vi "Get Tag.vi"(8 "error in (no error)":errorcluster, 11 "Item Configuration in":refnum<class "Item Configuration.lvclass">) -> (0 "error out":errorcluster, 2 "Project Info Tag":string, 3 "Item Configuration out":refnum<class "Item Configuration.lvclass">)   [LabVIEW 2013, in "Item Configuration.lvlib" / "Item Configuration.lvclass"]
uses:
  Item Configuration.lvclass
  Item Configuration.lvclass/Item Configuration.ctl
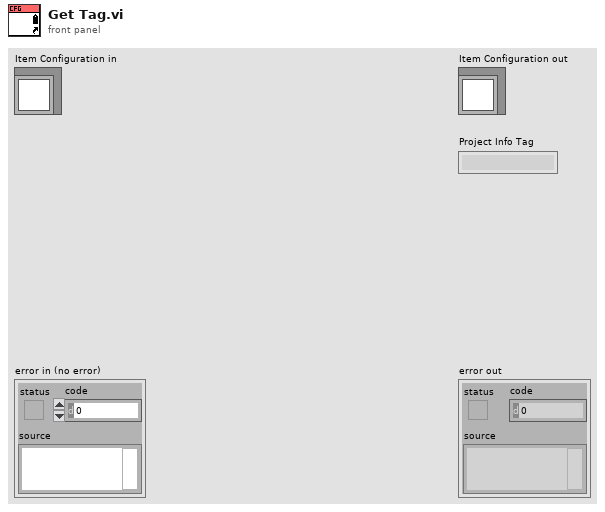
[diagram p1: front panel]
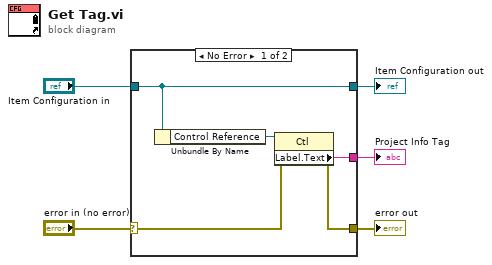
[diagram p0: block diagram]
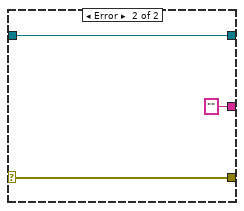
[diagram p2: hidden frame]
diagram:
  n1 = case shown="No Error" "error in (no error)" {
    selector: "error in (no error)" -> [w8 w13]
    tunnel: "Item Configuration in" -> [w6 w12]
    tunnel: [w9 "" ("Label.Text")] -> w4
    tunnel: [w7 w13] -> w2
    tunnel: [w6 w12] -> w1
    frame No Error {
      n2 = Unbundle By Name(w6) -> ("Control Reference"=w10:refnum<vi>)
      n3 = property class="Ctl"(reference=w10, error in=w8) -> (error out=w7:errorcluster, "Label.Text"=w9:string)  [unwired: 1 out]
    }
    frame Error {
    }
  }
  "error out" <- w2
  "Item Configuration out" <- w1
  "Project Info Tag" <- w4
